vi "Read.vi"(8 "error in (no error)":errorcluster, 11 "Xbox Controller in":refnum<class "Xbox Controller.lvclass">) -> (0 "error out":errorcluster, 1 "Velocity out":dbl, 2 "Direction out":cluster{dbl, dbl}, 4 "Stop?":bool, 5 "Boost?":bool)   [LabVIEW 2021, in "Xbox Controller.lvclass"]
doc: "MIT Licence\nCopyright (c) 2024 David Grollier"
uses:
  Xbox Controller.lvclass
  C:/Users/David/Documents/GameSoccerSpace/Source/Input Device/Input Device.lvclass
  Input Device.lvclass/Input Device.ctl
  Xbox Controller.lvclass/Xbox Controller.ctl
  <vilib>/Utility/inputDevices.llb/joystickAcquire.vi
  Input Device.lvclass
  Utils/Utils.lvlib
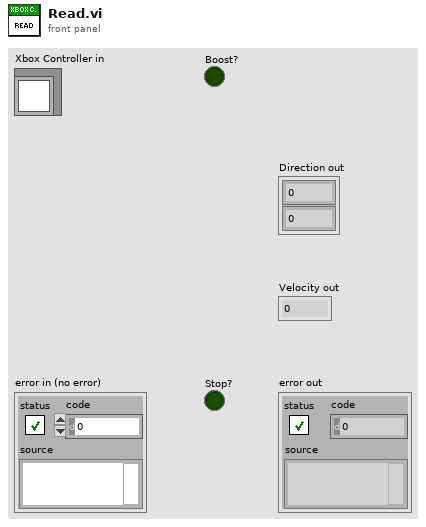
[diagram p1: front panel]
types:
  T1 = cluster{"X axis":i32, "Y axis":i32, "Z axis":i32, "X axis rotation":i32, "Y axis rotation":i32, "Z axis rotation":i32, "U axis":i32, "V axis":i32}
  T2 = cluster{"button 1":bool, "button 2":bool, "button 3":bool, "button 4":bool, "button 5":bool, "button 6":bool, "button 7":bool, "button 8":bool, "button 9":bool, "button 10":bool, "button 11":bool, "button 12":bool, "button 13":bool, "button 14":bool, "button 15":bool, "button 16":bool, "button 17":bool, "button 18":bool, "button 19":bool, "button 20":bool, "button 21":bool, "button 22":bool, "button 23":bool, "button 24":bool, "button 25":bool, "button 26":bool, "button 27":bool, "button 28":bool, "button 29":bool, "button 30":bool, "button 31":bool, "button 32":bool}
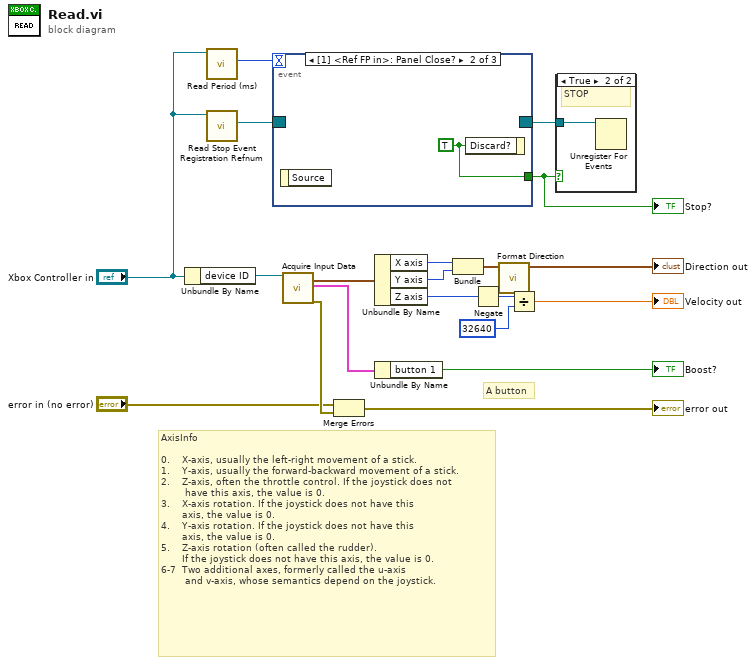
[diagram p0: block diagram]
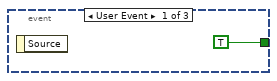
[diagram p3: hidden frame]
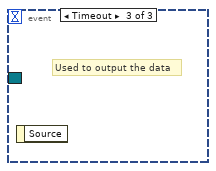
[diagram p4: hidden frame]
diagram:
  # "AxisInfo \n\n0.    X-axis, usually the left-right movement of a stick. \n1.    Y-axis, usually the forward-backward movement of a stick. \n2.    Z-axis, often the throttle control. If the joystick does not \n        have this axis, the value is 0. \n3.    X-axis rotation. If the joystick does not have this \n       axis, the value is 0. \n4.    Y-axis rotation. If the joystick does not have this \n       axis, the value is 0. \n5.    Z-axis rotation (often called the rudder). \n       If the joystick does not have this axis, the value is 0. \n6-7  Two additional axes, formerly called the u-axis\n        and v-axis, whose semantics depend on the joystick."
  # "A button"
  n1 = Unbundle By Name("Xbox Controller in") -> ("device ID"=w17:refnum<k1>)
  n2 = call "Read Period (ms).vi"("Input Device in"="Xbox Controller in") -> ("Period (ms)"=w19:i64)  [unwired: 10 in]
  n3 = call "Read Stop Event Registration Refnum.vi"("Input Device in"="Xbox Controller in") -> ("Stop Event Registration Refnum out"=w18:refnum<event-registration>)  [unwired: 10 in]
  n4 = event shown="[1] <Ref FP in>: Panel Close?" {
    selector: w18 -> [_ _ _]
    dyn-events: [_ _ _] -> w20
    timeout: w19 -> [_ _ _]
    tunnel: [TRUE w22 _] -> w6
    event User Event {
      n5 = event-data() -> ()  [unwired: 1 in, 1 out]
    }
    event Panel Close? {
      w22 = TRUE ("Discard?")
      n6 = event-data() -> ()  [unwired: 1 in, 1 out]
      n7 = event-data("Discard?"=w22) -> ()  [unwired: 1 in, 1 out]
    }
    event Timeout {
      # "Used to output the data"
      n8 = event-data() -> ()  [unwired: 1 in, 1 out]
    }
  }
  "Stop?" <- w6
  n9 = call-poly <vilib>:"Acquire Input Data.vi"("device ID"=w17) -> ("axis info"=w15:T1, "button info"=w16:T2, "error out"=w5:errorcluster)  [unwired: 14 in, 2 out]
  n10 = Merge Errors("error in (no error)", w5) -> (→"error out":errorcluster)
  n11 = Unbundle By Name(w15) -> ("X axis"=w13:i32, "Y axis"=w14:i32, "Z axis"=w8:i32)
  n12 = Unbundle By Name(w16) -> ("button 1"=→"Boost?":bool)
  n13 = Bundle("X axis"=w13, "Y axis"=w14) -> (w11:cluster{"X axis":i32, "Y axis":i32})  [unwired: 1 in]
  n14 = Negate(x=w8) -> (-x=w9:i32)
  n15 = call "Format Direction.vi"("Direction in"=w11) -> ("Formated Direction out"=→"Direction out":cluster{dbl, dbl})  [unwired: 10 in]
  n16 = Divide(x=w9, y=32640) -> (x/y=→"Velocity out":dbl)
  n17 = case shown="True" w6 {
    tunnel: w20 -> [_ w23]
    frame False {
      # "No Stop"
    }
    frame True {
      # "STOP"
      n18 = Unregister For Events(event registration refnum=w23) -> ()  [unwired: 1 in, 1 out]
    }
  }
